vi "_AttributeDataTypeError.vi"(1 "error in":errorcluster, 2 "location":string="[Unknown.vi]", 3 "user Data Type":T2=enum."UNKNOWN_DATA_TYPE", 4 "actual Data Type":T2=enum."UNKNOWN_DATA_TYPE", 5 "attribute name":string, 6 "device name":string) -> (0 "error out":errorcluster)   [LabVIEW 2014, in "tango.lvlib"]
uses:
  tango.lvlib
  Common VIs/Typedefs/_AttributeDataType_t.ctl
panel:
  out "LV Data Type Control":T1(ring)=enum."Unknown Data Type"
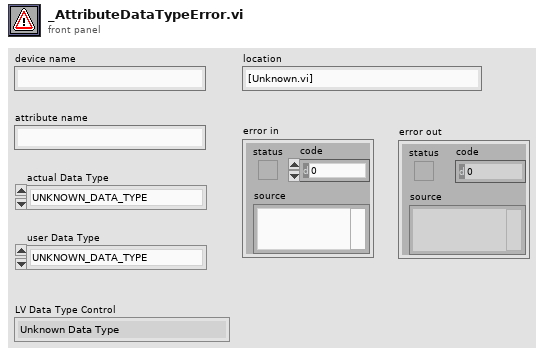
[diagram p1: front panel]
types:
  T1 = enum16{"State Scalar", "State Spectrum", "State Image", "String Scalar", "String Spectrum", "String Image", "Boolean Scalar", "Boolean Spectrum", "Boolean Image", "U8 Scalar", "U8 Spectrum", "U8 Image", "I16 Scalar", "I16 Spectrum", "I16 Image", "U16 Scalar", "U16 Spectrum", "U16 Image", "I32 Scalar", "I32 Spectrum", "I32 Image", "U32 Scalar", "U32 Spectrum  ", "U32 IMage", "I64 Scalar", "I64 Spectrum", "I64 Image", "U64 Scalar", "U64 Spectrum", "U64 Image ", "SGL Scalar", "SGL Spectrum", "SGL Image", "DBL Scalar", "DBL Spectrum", "DBL Image", "Unknown Data Type"}
  T2 = typedef "tango.lvlib/_AttributeDataType_t.ctl" = enum16{"STATE_SCA", "STATE_SPE", "STATE_IMG", "STRING_SCA", "STRING_SPE", "STRING_IMG", "BOOL_SCA", "BOOL_SPE", "BOOL_IMG", "UCHAR_SCA", "UCHAR_SPE", "UCHAR_IMG", "SHORT_SCA", "SHORT_SPE", "SHORT_IMG", "USHORT_SCA", "USHORT_SPE", "USHORT_IMG", "LONG_SCA", "LONG_SPE", "LONG_IMG", "ULONG_SCA", "ULONG_SPE", "ULONG_IMG", "LONG64_SCA", "LONG64_SPE", "LONG64_IMG", "ULONG64_SCA", "ULONG64_SPE", "ULONG64_IMG", "FLOAT_SCA", "FLOAT_SPE", "FLOAT_IMG", "DOUBLE_SCA", "DOUBLE_SPE", "DOUBLE_IMG", "UNKNOWN_DATA_TYPE"}
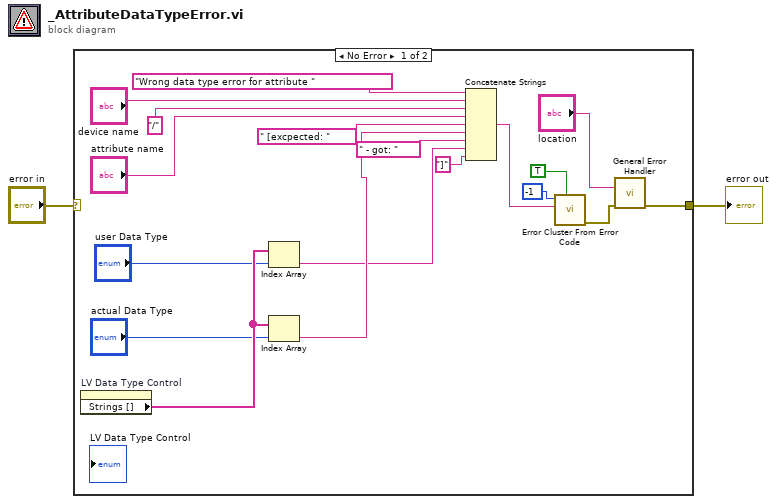
[diagram p0: block diagram]
diagram:
  n1 = case shown="No Error" "error in" {
    selector: "error in" -> [_ w21]
    tunnel: [w20 w21] -> w2
    frame No Error {
      n2 = property on="LV Data Type Control" class="Enum (strict)"() -> ("Strings []"=w12:string[])  [unwired: 2 in, 2 out]
      n3 = Index Array(array=w12, index="user Data Type") -> (element=w7:string)
      n4 = Index Array(array=w12, index="actual Data Type") -> (element=w8:string)
      n5 = Concatenate Strings("Wrong data type error for attribute " ("string"), "device name", "/" ("string"), "attribute name", " [excpected: " ("string"), w8, " - got: " ("string"), w7, "]" ("string")) -> (w6:string)
      n6 = call <vilib>:"Error Cluster From Error Code.vi"("show call chain? (False)"=TRUE, "error message (\"\")"=w6, "error code (0)"=-1) -> ("error out"=w4:errorcluster)  [unwired: 6 in]
      n7 = call <vilib>:"General Error Handler.vi"("[error source] (\" \")"="location", "error in (no error)"=w4) -> ("error out"=w20:errorcluster)  [unwired: 9 in, 4 out]
    }
    frame Error {
    }
  }
  "error out" <- w2
